vi "Pre Launch Init.vi"(11 "Elevator Controller in":refnum<class "Elevator Controller.lvclass">) -> (0 "error out":errorcluster, 3 "Elevator Controller out":refnum<class "Elevator Controller.lvclass">)   [LabVIEW 2019, in "Elevator Controller.lvlib" / "Elevator Controller.lvclass"]
doc: "(<B>Filename</B>: Actor Framework.lvlib:Actor.lvclass:Pre Launch Init.vi)\n\nDefines behavior that occurs after the Launch Nested Actor method is invoked but before the actor's Actor Core method begins running.\n\nBy default, this method does nothing. A descendant class may override it to define behavior."
uses:
  Elevator Controller.lvclass
  Elevator Controller.lvclass/Elevator Controller.ctl
  <vilib>/ActorFramework/Actor/Actor.lvclass
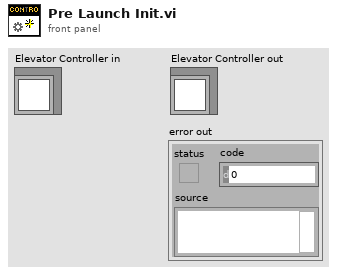
[diagram p1: front panel]
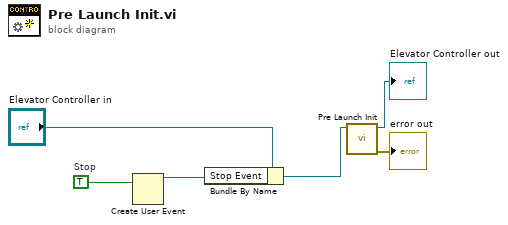
[diagram p0: block diagram]
diagram:
  w4 = TRUE  # Stop
  n1 = Create User Event(user event datatype=w4) -> (user event=w1:refnum<user-event>)  [unwired: 1 in, 1 out]
  n2 = Bundle By Name(cluster="Elevator Controller in", "Stop Event"=w1) -> (w2:refnum<class "Elevator Controller.lvclass">)
  n3 = call-parent "Pre Launch Init.vi"("Actor in"=w2) -> ("error out"=→"error out":errorcluster, "Actor out"=→"Elevator Controller out":refnum<class "Elevator Controller.lvclass">)  [unwired: 9 in]
